vi "fit_focus.vi"(8 "error in":errorcluster, 11 "Focus Measurements":cluster{"focus value":dbl, "height":dbl}[](array[cluster])) -> (0 "error out":errorcluster, 2 "error":dbl, 3 "focus height":dbl)   [LabVIEW 2011, in "gVision.lvlib"]
uses:
  gVision.lvlib
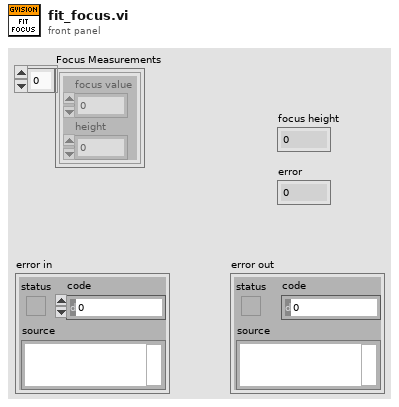
[diagram p1: front panel]
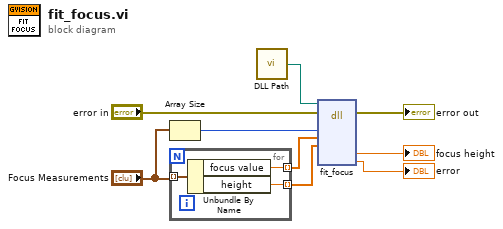
[diagram p0: block diagram]
diagram:
  n1 = Array Size(array="Focus Measurements") -> (size(s)=w1:i32)
  n2 = for {
    tunnel: "Focus Measurements" -> [w12] mode=indexing
    tunnel: [w11] -> w4 mode=indexing
    tunnel: [w10] -> w3 mode=indexing
    n3 = Unbundle By Name(w12) -> ("focus value"=w11:dbl, "height"=w10:dbl)
  }
  n4 = call "DLL Path.vi"() -> ("DLL Path"=w7:path)  [unwired: 5 in]
  n5 = dll-call lib="?" fn="fit_focus"(path in=w7, error in="error in", "num_measurements"=w1, "focus_values"=w4, "heights"=w3) -> (error out=→"error out":errorcluster, "mean"=→"focus height":dbl, "stdev"=→"error":dbl)  [unwired: 7 in, 1 out]
